vi "FSK.vi"() -> ()   [LabVIEW 2014]
uses:
  <vilib>/Analysis/8numeric.llb/1D Numeric Integration.vi
  <vilib>/measure/NI_MABase.lvlib
  <vilib>/Analysis/NI_AALPro.lvlib
panel:
  out "Waveform Chart 4":i16(graph)
  out "Waveform Chart 3":waveform(dbl)(graph)
  in  "amp 2":dbl format="%#_13g"
  in  "freq 3":dbl format="%#_13g"
  out "Waveform Chart 5":waveform(dbl)(graph)
  in  "Numeric 2":i32=1
  in  "freq 2":i32=1
  out "Waveform Chart 2":i16[](graph)
  in  "Numeric":i32=1
  in  "freq":i32=1
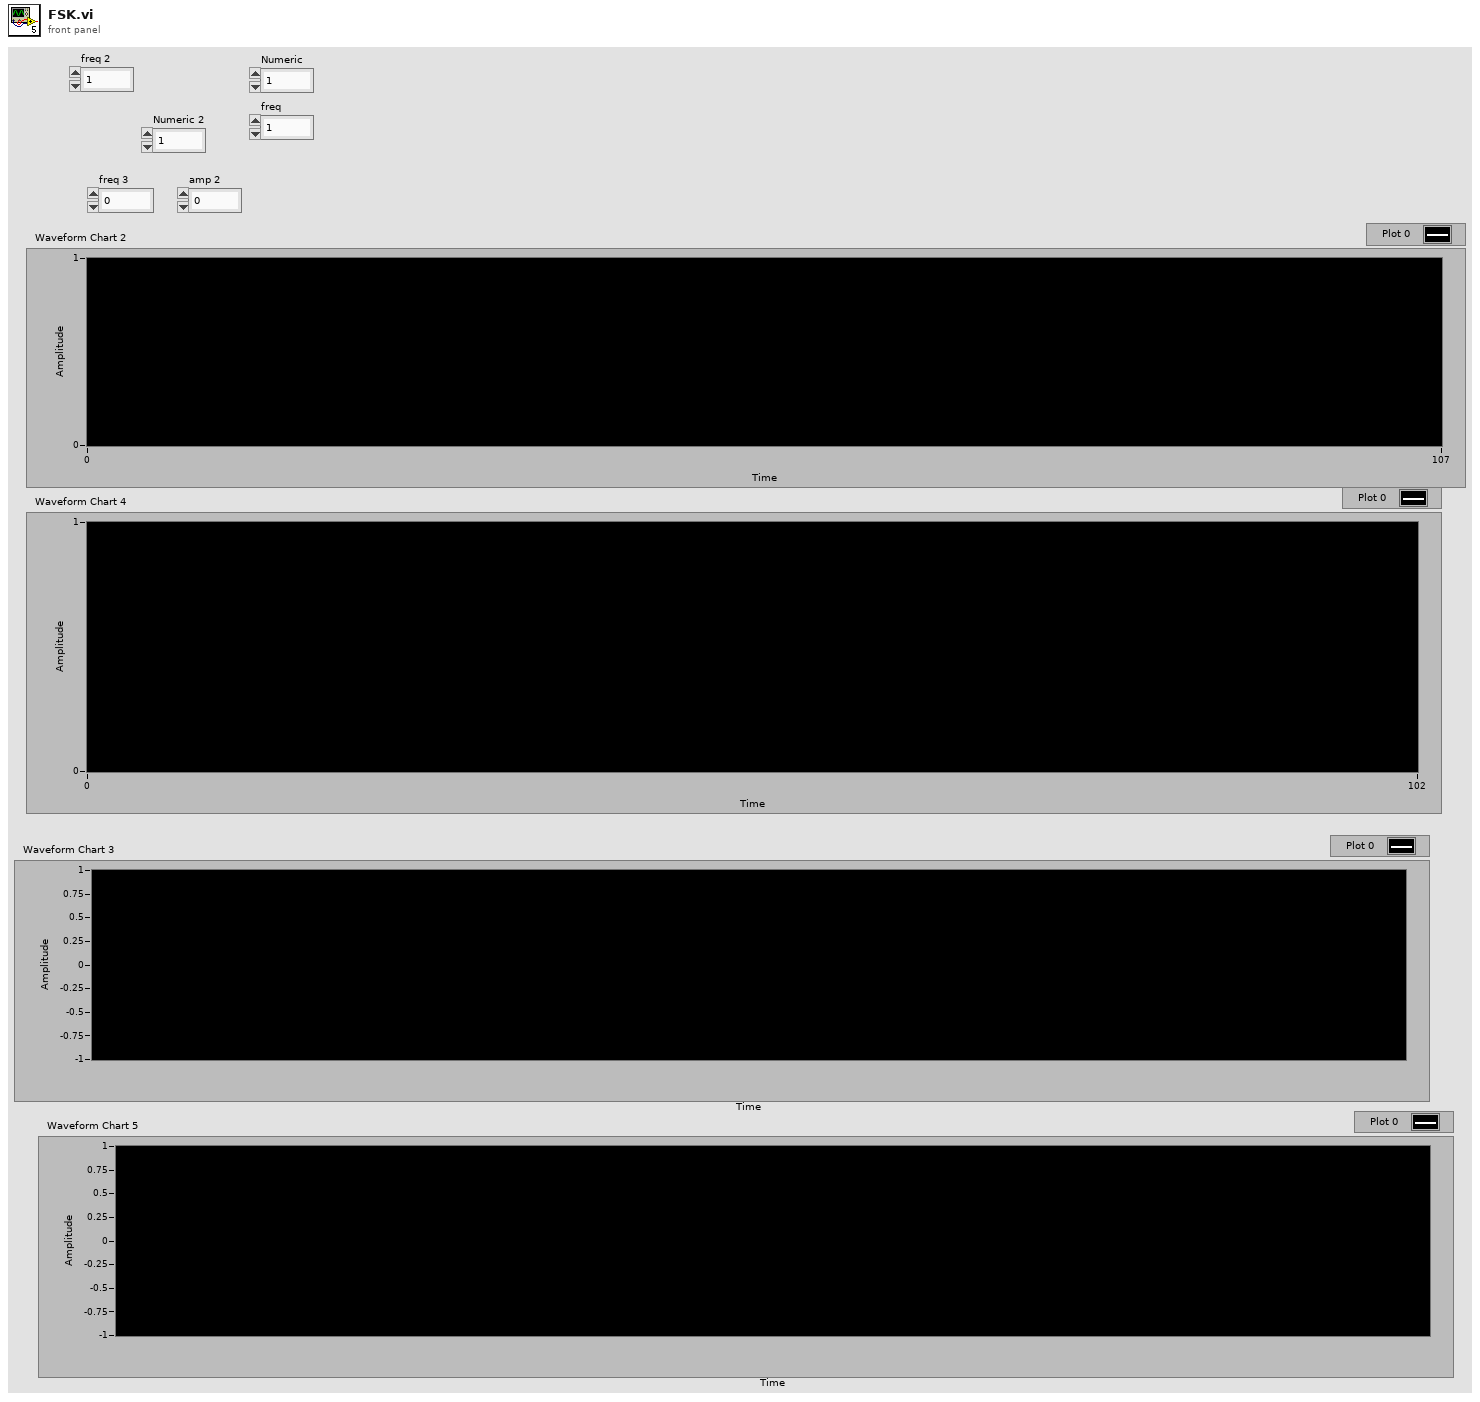
[diagram p1: front panel]
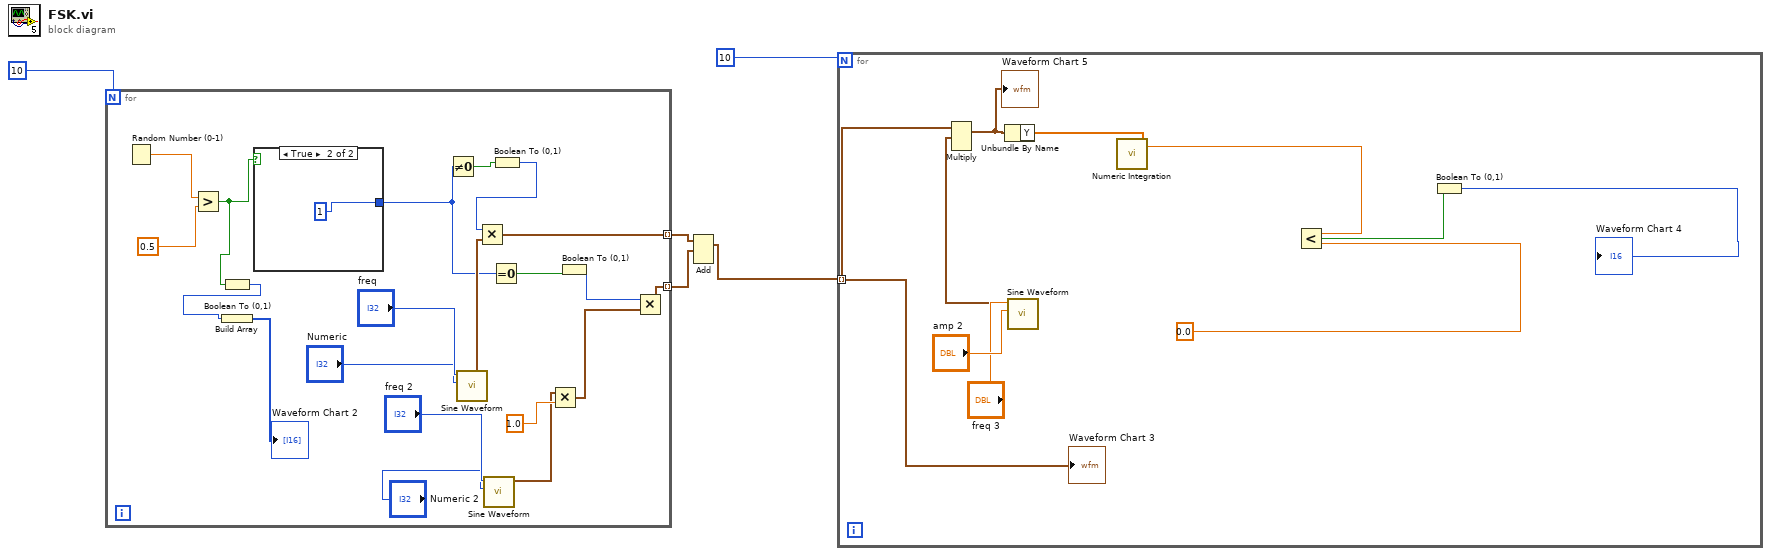
[diagram p0: block diagram]
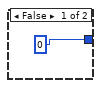
[diagram p2: hidden frame]
diagram:
  n1 = for {
    N: 10 ("Numeric") -> [_]
    tunnel: [w13] -> w4 mode=indexing
    tunnel: [w12] -> w3 mode=indexing
    n2 = Random Number (0-1)() -> (number: 0 to 1=w24:dbl)
    n3 = Greater?(x=w24, y=0.5) -> (0:w23:bool)
    n4 = Boolean To (0,1)(Boolean=w23) -> (0, 1=w22:i16)
    n5 = Build Array(w22) -> (→"Waveform Chart 2":i16[])
    n6 = case shown="True" w23 {
      tunnel: [0 1] -> w11
      frame False {
      }
      frame True {
      }
    }
    n7 = Not Equal To 0?(x=w11) -> (x != 0?=w19:bool)
    n8 = call <vilib>:"Sine Waveform.vi"("amplitude"="Numeric", "frequency"="freq") -> ("signal out"=w16:waveform(dbl))  [unwired: 8 in, 1 out]
    n9 = call <vilib>:"Sine Waveform.vi"("amplitude"="Numeric 2", "frequency"="freq 2") -> ("signal out"=w7:waveform(dbl))  [unwired: 8 in, 1 out]
    n10 = Equal To 0?(x=w11) -> (x = 0?=w17:bool)
    n11 = Boolean To (0,1)(Boolean=w19) -> (0, 1=w20:i16)
    n12 = Multiply(x=w20, y=w16) -> (x*y=w12:waveform(dbl))
    n13 = Multiply(x=w7, y=1.0) -> (x*y=w15:waveform(dbl))
    n14 = Boolean To (0,1)(Boolean=w17) -> (0, 1=w14:i16)
    n15 = Multiply(x=w14, y=w15) -> (x*y=w13:waveform(dbl))
  }
  n16 = Add(1:w4, 2:w3) -> (0:w2:waveform(dbl)[])  [unwired: 1 in, 1 out]
  n17 = for {
    N: 10 -> [_]
    tunnel: w2 -> [w30] mode=indexing
    n18 = call <vilib>:"Sine Waveform.vi"("amplitude"="amp 2", "frequency"="freq 3") -> ("signal out"=w29:waveform(dbl))  [unwired: 8 in, 1 out]
    n19 = Multiply(1:w29, 2:w30) -> (0:w28:waveform(dbl))  [unwired: 1 in, 1 out]
    "Waveform Chart 5" <- w28
    n20 = Unbundle By Name(w28) -> ("Y"=w34:dbl[])
    n21 = call-poly <vilib>:"Numeric Integration.vi"("Input Array"=w34) -> ("result"=w37:dbl)  [unwired: 2 in, 1 out]
    n22 = Less?(x=w37, y=0.0) -> (x < y?=w35:bool)
    n23 = Boolean To (0,1)(Boolean=w35) -> (0, 1=→"Waveform Chart 4":i16)
    "Waveform Chart 3" <- w30
  }
